vi "Test - 5.vi"() -> ()   [LabVIEW 2013]
uses:
  Section/Section.lvclass
  Channel/Ctls/ChannelSetting.ctl
  Channel/Ctls/IOType.ctl
  Channel/Ctls/Dimensions.ctl
  Generic/Generic.lvclass
  Channel/Channel.lvclass
  Item/Item.lvclass
  <vilib>/NI Veristand/Custom Device API/Custom Device API.lvlib
panel:
  out "PathName 3":string
  in  "PathName 2":string="Root/Section1"
  out "数组":string[](array[string])
  out "Found":bool
  out "PathName":string
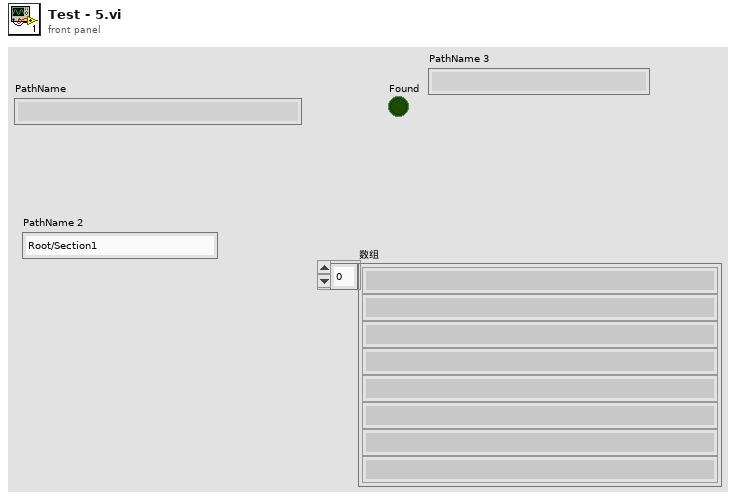
[diagram p1: front panel]
types:
  T1 = typedef "Hierarchy Framework.lvlib/Channel.lvclass/ChannelSetting.ctl" = cluster{"IOType":T2, "DefaultValue":dbl[][], "Dimensions":T3, "Units":string, "Description":string, "Faultable":bool}
  T2 = typedef "Hierarchy Framework.lvlib/Channel.lvclass/IOType.ctl" = enum16{"Input", "Output"}
  T3 = typedef "Hierarchy Framework.lvlib/Channel.lvclass/Dimensions.ctl" = cluster{"Row":i32, "Column":i32}
  T4 = typedef "Hierarchy Framework.lvlib/Item.lvclass/Item Reference.ctl" = u64
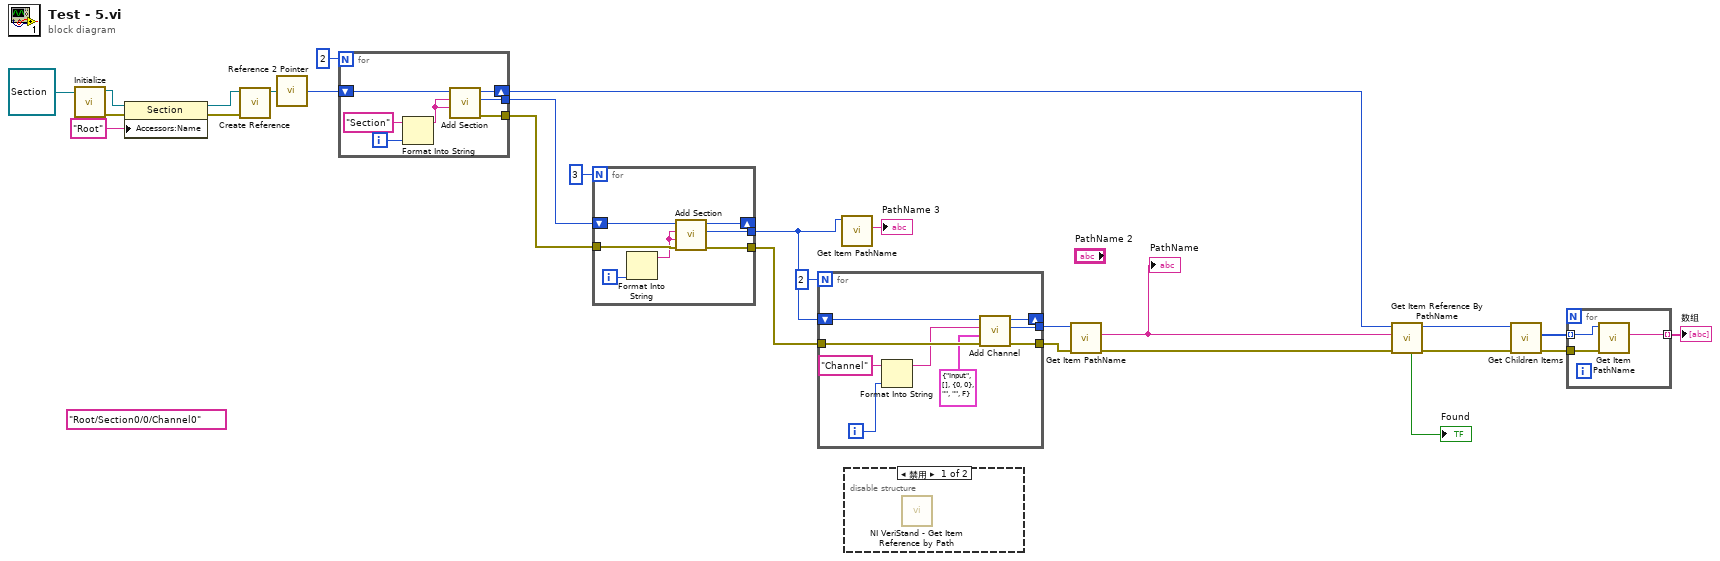
[diagram p0: block diagram]
diagram:
  (unwired) "Root/Section0/0/Channel0" ("Name")
  n1 = call-dynamic "Initialize.vi"("Section输入"=refnum<class "Section.lvclass"> refnum ("Framework.lvlib:Section")) -> ("error out"=w24:errorcluster, "Section输出"=w27:refnum<class "Section.lvclass">)  [unwired: 9 in]
  n2 = property class="Section"(reference=w27, error in=w24, "Accessors:Name"="Root" ("Name")) -> (reference out=w26:refnum<class "Section.lvclass">, error out=w21:errorcluster)
  n3 = call "Create Reference.vi"("error in (no error)"=w21, "Generic"=w26) -> ("Generic Reference"=w23:refnum<data-value>)  [unwired: 8 in, 1 out]
  n4 = call "Reference 2 Pointer.vi"("Generic Reference"=w23) -> ("Pointer"=w20:u64)  [unwired: 1 out]
  n5 = for {
    N: 2 -> [_]
    shift-right: [w33] -> w16
    shift-left: w20 -> [w34]
    tunnel: [w30] -> w18
    tunnel: [w29] -> w15
    i -> [w32]
    n6 = Format Into String(initial string="Section" ("初始字符串"), w32) -> (resulting string=w28:string)  [unwired: 2 in, 1 out]
    n7 = call "Add Section.vi"("TypeGUID"=w28, "SectionName"=w28, "Section Reference in"=w34) -> ("error out"=w29:errorcluster, "Section Reference"=w30:u64, "Section Reference out"=w33:u64)  [unwired: 5 in, 1 out]
  }
  n8 = for {
    N: 3 -> [_]
    shift-right: [w40] -> _
    shift-left: w18 -> [w41]
    tunnel: [w38] -> w2
    tunnel: w15 -> [w37]
    tunnel: [w36] -> w14
    i -> [w39]
    n9 = Format Into String(w39) -> (resulting string=w35:string)  [unwired: 3 in, 1 out]
    n10 = call "Add Section.vi"("error in (no error)"=w37, "TypeGUID"=w35, "SectionName"=w35, "Section Reference in"=w41) -> ("error out"=w36:errorcluster, "Section Reference"=w38:u64, "Section Reference out"=w40:u64)  [unwired: 4 in, 1 out]
  }
  n11 = for {
    N: 2 -> [_]
    tunnel: w14 -> [w49]
    shift-right: [w48] -> _
    shift-left: w2 -> [w50]
    tunnel: [w43] -> w11
    tunnel: [w42] -> w12
    i -> [w46]
    n12 = Format Into String(initial string="Channel" ("初始字符串"), w46) -> (resulting string=w44:string)  [unwired: 2 in, 1 out]
    n13 = call "Add Channel.vi"("error in (no error)"=w49, "Channel Setting"=T1 {"IOType"=enum."Input", "DefaultValue"=[], "Dimensions"={"Row"=0, "Column"=0}, "Units"="", "Description"="", "Faultable"=FALSE}, "Channel Name"=w44, "Section Reference in"=w50) -> ("error out"=w43:errorcluster, "Channel Reference"=w42:u64, "Section Reference out"=w48:u64)  [unwired: 4 in, 1 out]
  }
  n14 = call "Get Item PathName.vi"("Item Reference in"=w2) -> ("PathName"=→"PathName 3":string)  [unwired: 7 in, 3 out]
  n15 = disable-structure shown="禁用" {
    frame Disabled {
      n16 = call <vilib>:"NI VeriStand - Get Item Reference by Path.vi"() -> ()  [unwired: 8 in, 4 out]
    }
    frame Enabled {
    }
  }
  n17 = call "Get Item PathName.vi"("error in (no error)"=w11, "Item Reference in"=w12) -> ("error out"=w10:errorcluster, "PathName"=w8:string)  [unwired: 6 in, 2 out]
  "PathName" <- w8
  n18 = call "Get Item Reference By PathName.vi"("error in (no error)"=w10, "Item PathName"=w8, "Root Item Reference in"=w16) -> ("error out"=w6:errorcluster, "Root Item Reference out"=w7:T4, "found"=→"Found":bool)  [unwired: 5 in, 1 out]
  n19 = call "Get Children Items.vi"("error in (no error)"=w6, "Section Reference in"=w7) -> ("error out"=w4:errorcluster, "Children Item References"=w5:u64[])  [unwired: 5 in, 3 out]
  n20 = for {
    tunnel: w5 -> [w53] mode=indexing
    tunnel: w4 -> [w52]
    tunnel: [w51] -> w3 mode=indexing
    n21 = call "Get Item PathName.vi"("error in (no error)"=w52, "Item Reference in"=w53) -> ("PathName"=w51:string)  [unwired: 6 in, 3 out]
  }
  "数组" <- w3
